vi "TUNA RT main.vi"() -> ()   [LabVIEW 2014]
uses:
  <vilib>/myRIO/Instrument Drivers/Onboard IO/PWM/typedefs/PWM Reference.ctl
  <vilib>/myRIO/Common/Instrument Driver Framework/Utilities/typedefs/myRIO Generic Hardware Reference.ctl
  <vilib>/myRIO/Common/Instrument Driver Framework/Utilities/typedefs/Hardware Version Enum.ctl
  <vilib>/myRIO/Common/Instrument Driver Framework/Utilities/typedefs/myRIO v1.0 Reference.ctl
  <vilib>/myRIO/Common/Instrument Driver Framework/Utilities/typedefs/Generic FPGA Reference.ctl
  <vilib>/myRIO/Common/Instrument Driver Framework/myRIO v1.0/PWM/typedefs/PWM Channels Enum.ctl
  <vilib>/myRIO/Instrument Drivers/Onboard IO/PWM/typedefs/PWM Configuration.ctl
  <vilib>/userdefined/High Color/nirio_resource_hc.ctl
  <vilib>/myRIO/Instrument Drivers/Onboard IO/DIO/typedefs/DIO Reference.ctl
  <vilib>/myRIO/Common/Instrument Driver Framework/myRIO v1.0/DIO/typedefs/DIO Channels List.ctl
  <vilib>/myRIO/Common/Instrument Driver Framework/myRIO v1.0/DIO/typedefs/DIO Channels Enum.ctl
  <vilib>/myRIO/Instrument Drivers/Onboard IO/AI/typedefs/AI Reference.ctl
  <vilib>/myRIO/Common/Instrument Driver Framework/myRIO v1.0/AI/typedefs/AI Channels List.ctl
  <vilib>/myRIO/Common/Instrument Driver Framework/myRIO v1.0/AI/typedefs/AI Channels Enum.ctl
  <vilib>/myRIO/Common/Instrument Driver Framework/Utilities/typedefs/Analog Scaling Constants List.ctl
  <vilib>/myRIO/Common/Instrument Driver Framework/Utilities/typedefs/Analog Scaling Constants.ctl
  <vilib>/Instr/_visa.llb/VISA Flush IO Buffer Mask.ctl
  <vilib>/myRIO/Common/Instrument Driver Framework/myRIO v1.0/PWM/vis/myRIO v1.1 Open PWM.vi
  <vilib>/myRIO/Common/Instrument Driver Framework/myRIO v1.0/DIO/vis/myRIO v1.1 Open DIO.vi
  <vilib>/myRIO/Common/Instrument Driver Framework/myRIO v1.0/AI/vis/myRIO v1.1 Open AI.vi
  <vilib>/myRIO/Common/Instrument Driver Framework/Utilities/vis/Validate Channels.vi
  <vilib>/myRIO/Common/Instrument Driver Framework/myRIO v1.0/PWM/vis/myRIO v1.0 Reserve PWM.vi
  <vilib>/myRIO/Common/Instrument Driver Framework/myRIO v1.0/DIO/vis/myRIO v1.0 Reserve DIO.vi
  <vilib>/myRIO/Common/Instrument Driver Framework/myRIO v1.0/AI/vis/myRIO v1.0 Reserve AI.vi
  <vilib>/myRIO/Common/Instrument Driver Framework/myRIO v1.0/AI/vis/myRIO v1.0 Close AI.vi
  <vilib>/myRIO/Common/Instrument Driver Framework/myRIO v1.0/DIO/vis/myRIO v1.0 Close DIO.vi
  <vilib>/myRIO/Common/Instrument Driver Framework/myRIO v1.0/PWM/vis/myRIO v1.0 Close PWM.vi
  <vilib>/myRIO/Common/Instrument Driver Framework/myRIO v1.0/PWM/vis/myRIO v1.0 Build MUX Configuration PWM.vi
  <vilib>/myRIO/Common/Instrument Driver Framework/myRIO v1.0/Resource Manager/vis/myRIO v1.0 Reserve Channel List.vi
  <vilib>/myRIO/Common/Instrument Driver Framework/myRIO v1.0/DIO/vis/myRIO v1.0 Build MUX Configuration DIO.vi
  <vilib>/myRIO/Common/Instrument Driver Framework/myRIO v1.0/AI/vis/myRIO v1.0 Build MUX Configuration AI.vi
  <vilib>/myRIO/Common/Instrument Driver Framework/myRIO v1.0/AI/vis/myRIO v1.0 Unreserve AI.vi
  <vilib>/myRIO/Common/Instrument Driver Framework/myRIO v1.0/DIO/vis/myRIO v1.0 Unreserve DIO.vi
  <vilib>/myRIO/Common/Instrument Driver Framework/myRIO v1.0/PWM/vis/myRIO v1.0 Unreserve PWM.vi
  <vilib>/myRIO/Common/Instrument Driver Framework/myRIO v1.0/Resource Manager/vis/myRIO v1.0 Create Configuration List.vi
  <vilib>/myRIO/Common/Instrument Driver Framework/myRIO v1.0/Resource Manager/vis/myRIO v1.0 Reserve Channel.vi
  <vilib>/myRIO/Common/Instrument Driver Framework/myRIO v1.0/Resource Manager/vis/myRIO v1.0 Unreserve Channel.vi
  <vilib>/myRIO/Common/Instrument Driver Framework/myRIO v1.0/Resource Manager/vis/myRIO v1.0 Unreserve Channel List.vi
  <vilib>/myRIO/Common/Instrument Driver Framework/myRIO v1.0/Resource Manager/vis/myRIO v1.0 Build Mutex Name.vi
  <vilib>/Utility/VariantDataType/GetNumericInfo.vi
  <vilib>/Utility/error.llb/Error Cluster From Error Code.vi
  <vilib>/myRIO/Common/Instrument Driver Framework/myRIO v1.0/myRIO v1.1 Open.vi
  <vilib>/myRIO/Common/Instrument Driver Framework/myRIO v1.0/AI/vis/myRIO v1.0 Get Scaling Constants AI.vi
  <vilib>/myRIO/Common/Instrument Driver Framework/Utilities/vis/IO Manager.vi
  <vilib>/myRIO/Common/Instrument Driver Framework/Utilities/vis/Configuration Manager.vi
  <vilib>/myRIO/Common/Instrument Driver Framework/myRIO v1.0/myRIO v1.0 Close.vi
  <vilib>/myRIO/Common/Instrument Driver Framework/myRIO v1.0/Resource Manager/vis/myRIO v1.0 Configure IO.vi
  <vilib>/myRIO/Common/Instrument Driver Framework/myRIO v1.0/AI/vis/myRIO v1.0 Read AI.vi
  <vilib>/myRIO/Common/Instrument Driver Framework/myRIO v1.0/DIO/vis/myRIO v1.0 Write DIO.vi
  <vilib>/myRIO/Common/Instrument Driver Framework/myRIO v1.0/PWM/vis/myRIO v1.0 Write PWM.vi
  <vilib>/myRIO/Common/Instrument Driver Framework/myRIO v1.0/DIO/vis/myRIO v1.0 Shutdown DIO.vi
  <vilib>/myRIO/Common/Instrument Driver Framework/myRIO v1.0/PWM/vis/myRIO v1.0 Shutdown PWM.vi
  <vilib>/myRIO/Instrument Drivers/Onboard IO/AI/vis/myRIO AI Open.xnode
  <vilib>/myRIO/Instrument Drivers/Onboard IO/DIO/vis/myRIO DIO Open.xnode
  <vilib>/myRIO/Instrument Drivers/Onboard IO/PWM/vis/myRIO PWM Open.xnode
  <vilib>/myRIO/Instrument Drivers/Onboard IO/AI/AI.lvlib
  <vilib>/myRIO/Instrument Drivers/Onboard IO/DIO/DIO.lvlib
  <vilib>/myRIO/Instrument Drivers/Onboard IO/PWM/PWM.lvlib
panel:
  in  "Tab Control":T1(tab)
  out "GLED":bool
  out "BLED":bool
  out "RLED":bool
  in  "stop":bool
  out "Midbrain?":bool
  out "Rudder":dbl(knob) min=-45.0 max=45.0 step=1.0 scale=-45.0..45.0
  out "Speed":dbl(knob) min=-9.0 max=9.0 step=1.0 scale=-50.0..50.0
  out "Hindbrain?":bool
  out "Forebrain?":bool
  out "Battery Dead?":bool
  out "Complete?":bool=TRUE
  out "Arbiter Graph":cluster{dbl, dbl, dbl[]}(graph)
  out "GPS Time Out?":bool
  in  "Run?":bool
  in  "MSpeed":dbl(slide) scale=-50.0..50.0 scale format="%#.1g"
  in  "MHeading":dbl(slide) scale=-180.0..180.0 scale format="%_1f"
  in  "Manual?":bool
  out "Camera Data":T2(array[cluster])
  out "Boat Status":T3={"GPS"={"X pos"=0, "Y pos"=0, "Heading"=0.0}, "IR Sensors"=[{"Name"="Bow", "Angle"=0.0, "Distance"=0.0}], "MOT BAT"=7.2, "RIO BAT"=7.2}
  out "Act Com":T4
  out "Forebrain ACT":dbl[](array[numeric])
  out "IR Sensors":T5(array[cluster])
  out "GPS":cluster{"X pos":i32, "Y pos":i32, "Heading":dbl}
  out "RED LED":bool
  out "GREEN LED":bool
  out "BLUE LED":bool
  in  "MDF":T6(array[cluster])=[{"Type"=enum."Start", "X"=250, "Y"=250, "Speed"=0, "Behaviors"=enum."Open Water Transit"}, {"Type"=enum."Waypoint", "X"=400, "Y"=100, "Speed"=20, "Behaviors"=enum."P-Wall Follow"}, {"Type"=enum."Waypoint", "X"=250, "Y"=250, "Speed"=20, "Behaviors"=enum."Open Water Transit"}, {"Type"=enum."Waypoint", "X"=250, "Y"=400, "Speed"=20, "Behaviors"=enum."Open Water Transit"}, {"Type"=enum."Waypoint", "X"=100, "Y"=400, "Speed"=20, "Behaviors"=enum."Open Water Transit"}, {"Type"=enum."End", "X"=250, "Y"=250, "Speed"=0, "Behaviors"=enum."Open Water Transit"}]
  in  "TUNA\nTAG":string="C"
  in  "GPS\nerror in":errorcluster
  in  "GPS\nVISA resource name":refnum<visa-resource-name>="ASRL2::INSTR"
  in  "Comms\nVISA resource name":refnum<visa-resource-name>="ASRL1::INSTR"
  in  "Comms\nerror in":errorcluster
  out "Invalid Pos?":bool
  out "error out":errorcluster
  out "Forebrain Comd":T7
  out "Debug IR \nRaw Readings":T5(array[cluster])
  out "Comms\nHandshake?":bool
  out "GPS \nHandshake?":bool
  out "Ready to execute handshake":bool
  out "size(s)":i32
  out "MDF Active":T6(array[cluster])
  # "BEHAVIOR LIGHTS"
  # "To start the Tug, press the \">\" key in the tool bar.\n\nPress the Run? control to start the Mission.\n\nWhen complete the Complete? indicator will light.\n\nIf the Run? is not pressed again, the mission will start again.\n\nAlways press the STOP button to end the operation!!!!!!!!!!!!!"
  # "Press the Manual? button to control\nthe Tug from the sliders"
  # "Stuck indicates that\nthe boat is not moving."
  # "Enter the Letter\nof  your Tug"
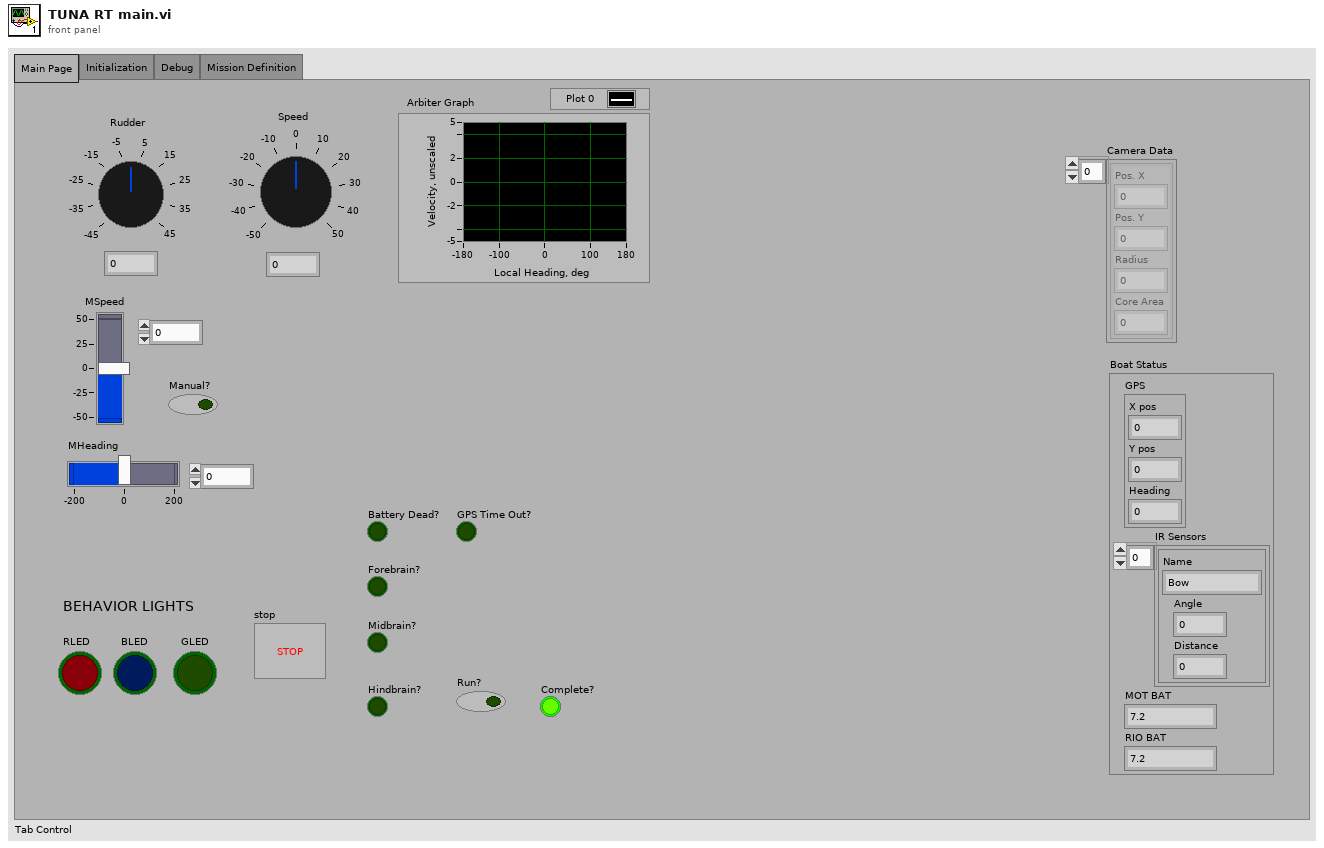
[diagram p1: front panel]
types:
  T1 = enum32{"Main Page", "Initialization", "Debug", "Mission Definition"}
  T2 = cluster{"Pos. X":i32, "Pos. Y":i32, "Radius":i32, "Core Area":i32}[]
  T3 = cluster{"GPS":cluster{"X pos":i32, "Y pos":i32, "Heading":dbl}, "IR Sensors":cluster{"Name":string, "Angle":dbl, "Distance":dbl}[], "MOT BAT":dbl, "RIO BAT":dbl}
  T4 = cluster{"Desired Local\nHeading":dbl, "Desired\nSpeed":dbl}
  T5 = cluster{"Name":string, "Angle":dbl, "Distance":dbl}[]
  T6 = cluster{"Type":enum16{"Start", "Waypoint", "End"}, "X":i32, "Y":i32, "Speed":i32, "Behaviors":enum16{"Open Water Transit", "P-Wall Follow", "S-Wall Follow", "Dock"}}[]
  T7 = cluster{"Behaviors":enum16{"Open Water Transit", "P-Wall Follow", "S-Wall Follow", "Dock"}, "Behavior\nVelocity":dbl}
  T8 = typedef "nirio_resource_hc.ctl" = tag
  T9 = typedef "Hardware Version Enum.ctl" = enum16{"Unknown", "myRIO-1900", "myRIO-1950"}
  T10 = enum16{"Open Water Transit", "P-Wall Follow", "S-Wall Follow", "Dock"}
  T11 = typedef "PWM.lvlib/PWM Reference.ctl" = cluster{"myRIO Reference":T12, "PWM Channels Enum":T15, "PWM Configuration":T16}
  T12 = typedef "myRIO Generic Hardware Reference.ctl" = cluster{"myRIO Model":T9, "myRIO Hardware Reference":T13}
  T13 = typedef "myRIO v1.0 Reference.ctl" = cluster{"Generic FPGA Reference":T14, "Allow multiple opens":bool}
  T14 = typedef "Generic FPGA Reference.ctl" = refnum<k20>
  T15 = typedef "PWM Channels Enum.ctl" = enum16{"Not Connected", "C/PWM0", "C/PWM1", "A/PWM0", "A/PWM1", "A/PWM2", "B/PWM0", "B/PWM1", "B/PWM2"}
  T16 = typedef "PWM.lvlib/PWM Configuration.ctl" = cluster{"Frequency":dbl, "Duty Cycle":dbl}
  T17 = typedef "DIO.lvlib/DIO Reference.ctl" = cluster{"myRIO Reference":T12, "DIO Channels List":T18}
  T18 = typedef "DIO Channels List.ctl" = T19[]
  T19 = typedef "DIO Channels Enum.ctl" = enum16{"Not Connected", "C/DIO0", "C/DIO1", "C/DIO2", "C/DIO3", "C/DIO4", "C/DIO5", "C/DIO6", "C/DIO7", "A/DIO0", "A/DIO1", "A/DIO2", "A/DIO3", "A/DIO4", "A/DIO5", "A/DIO6", "A/DIO7", "A/DIO8", "A/DIO9", "A/DIO10", "A/DIO11", "A/DIO12", "A/DIO13", "A/DIO14", "A/DIO15", "B/DIO0", "B/DIO1", "B/DIO2", "B/DIO3", "B/DIO4", "B/DIO5", "B/DIO6", "B/DIO7", "B/DIO8", "B/DIO9", "B/DIO10", "B/DIO11", "B/DIO12", "B/DIO13", "B/DIO14", "B/DIO15", "LED0", "LED1", "LED2", "LED3", "Button0"}
  T20 = typedef "AI.lvlib/AI Reference.ctl" = cluster{"myRIO Reference":T12, "AI Channels List":T21, "AI Scaling Constants List":T23}
  T21 = typedef "AI Channels List.ctl" = T22[]
  T22 = typedef "AI Channels Enum.ctl" = enum16{"Not Connected", "AudioIn/Left", "AudioIn/Right", "C/AI0", "C/AI1", "A/AI0", "A/AI1", "A/AI2", "A/AI3", "B/AI0", "B/AI1", "B/AI2", "B/AI3"}
  T23 = typedef "Analog Scaling Constants List.ctl" = T24[]
  T24 = typedef "Analog Scaling Constants.ctl" = cluster{"LSB Weight (Volts)":dbl, "Offset (Volts)":dbl, "Signed?":bool}
  T25 = cluster{"Obs Avoid Array":dbl[], "P-Wall Array":dbl[], "S-Wall Array":dbl[], "Unstuck Array":dbl[]}
  T26 = typedef "VISA Flush IO Buffer Mask.ctl" = u16
  T27 = cluster{"Behaviors":enum16{"Open Water Transit", "P-Wall Follow", "S-Wall Follow", "Dock"}, dbl}
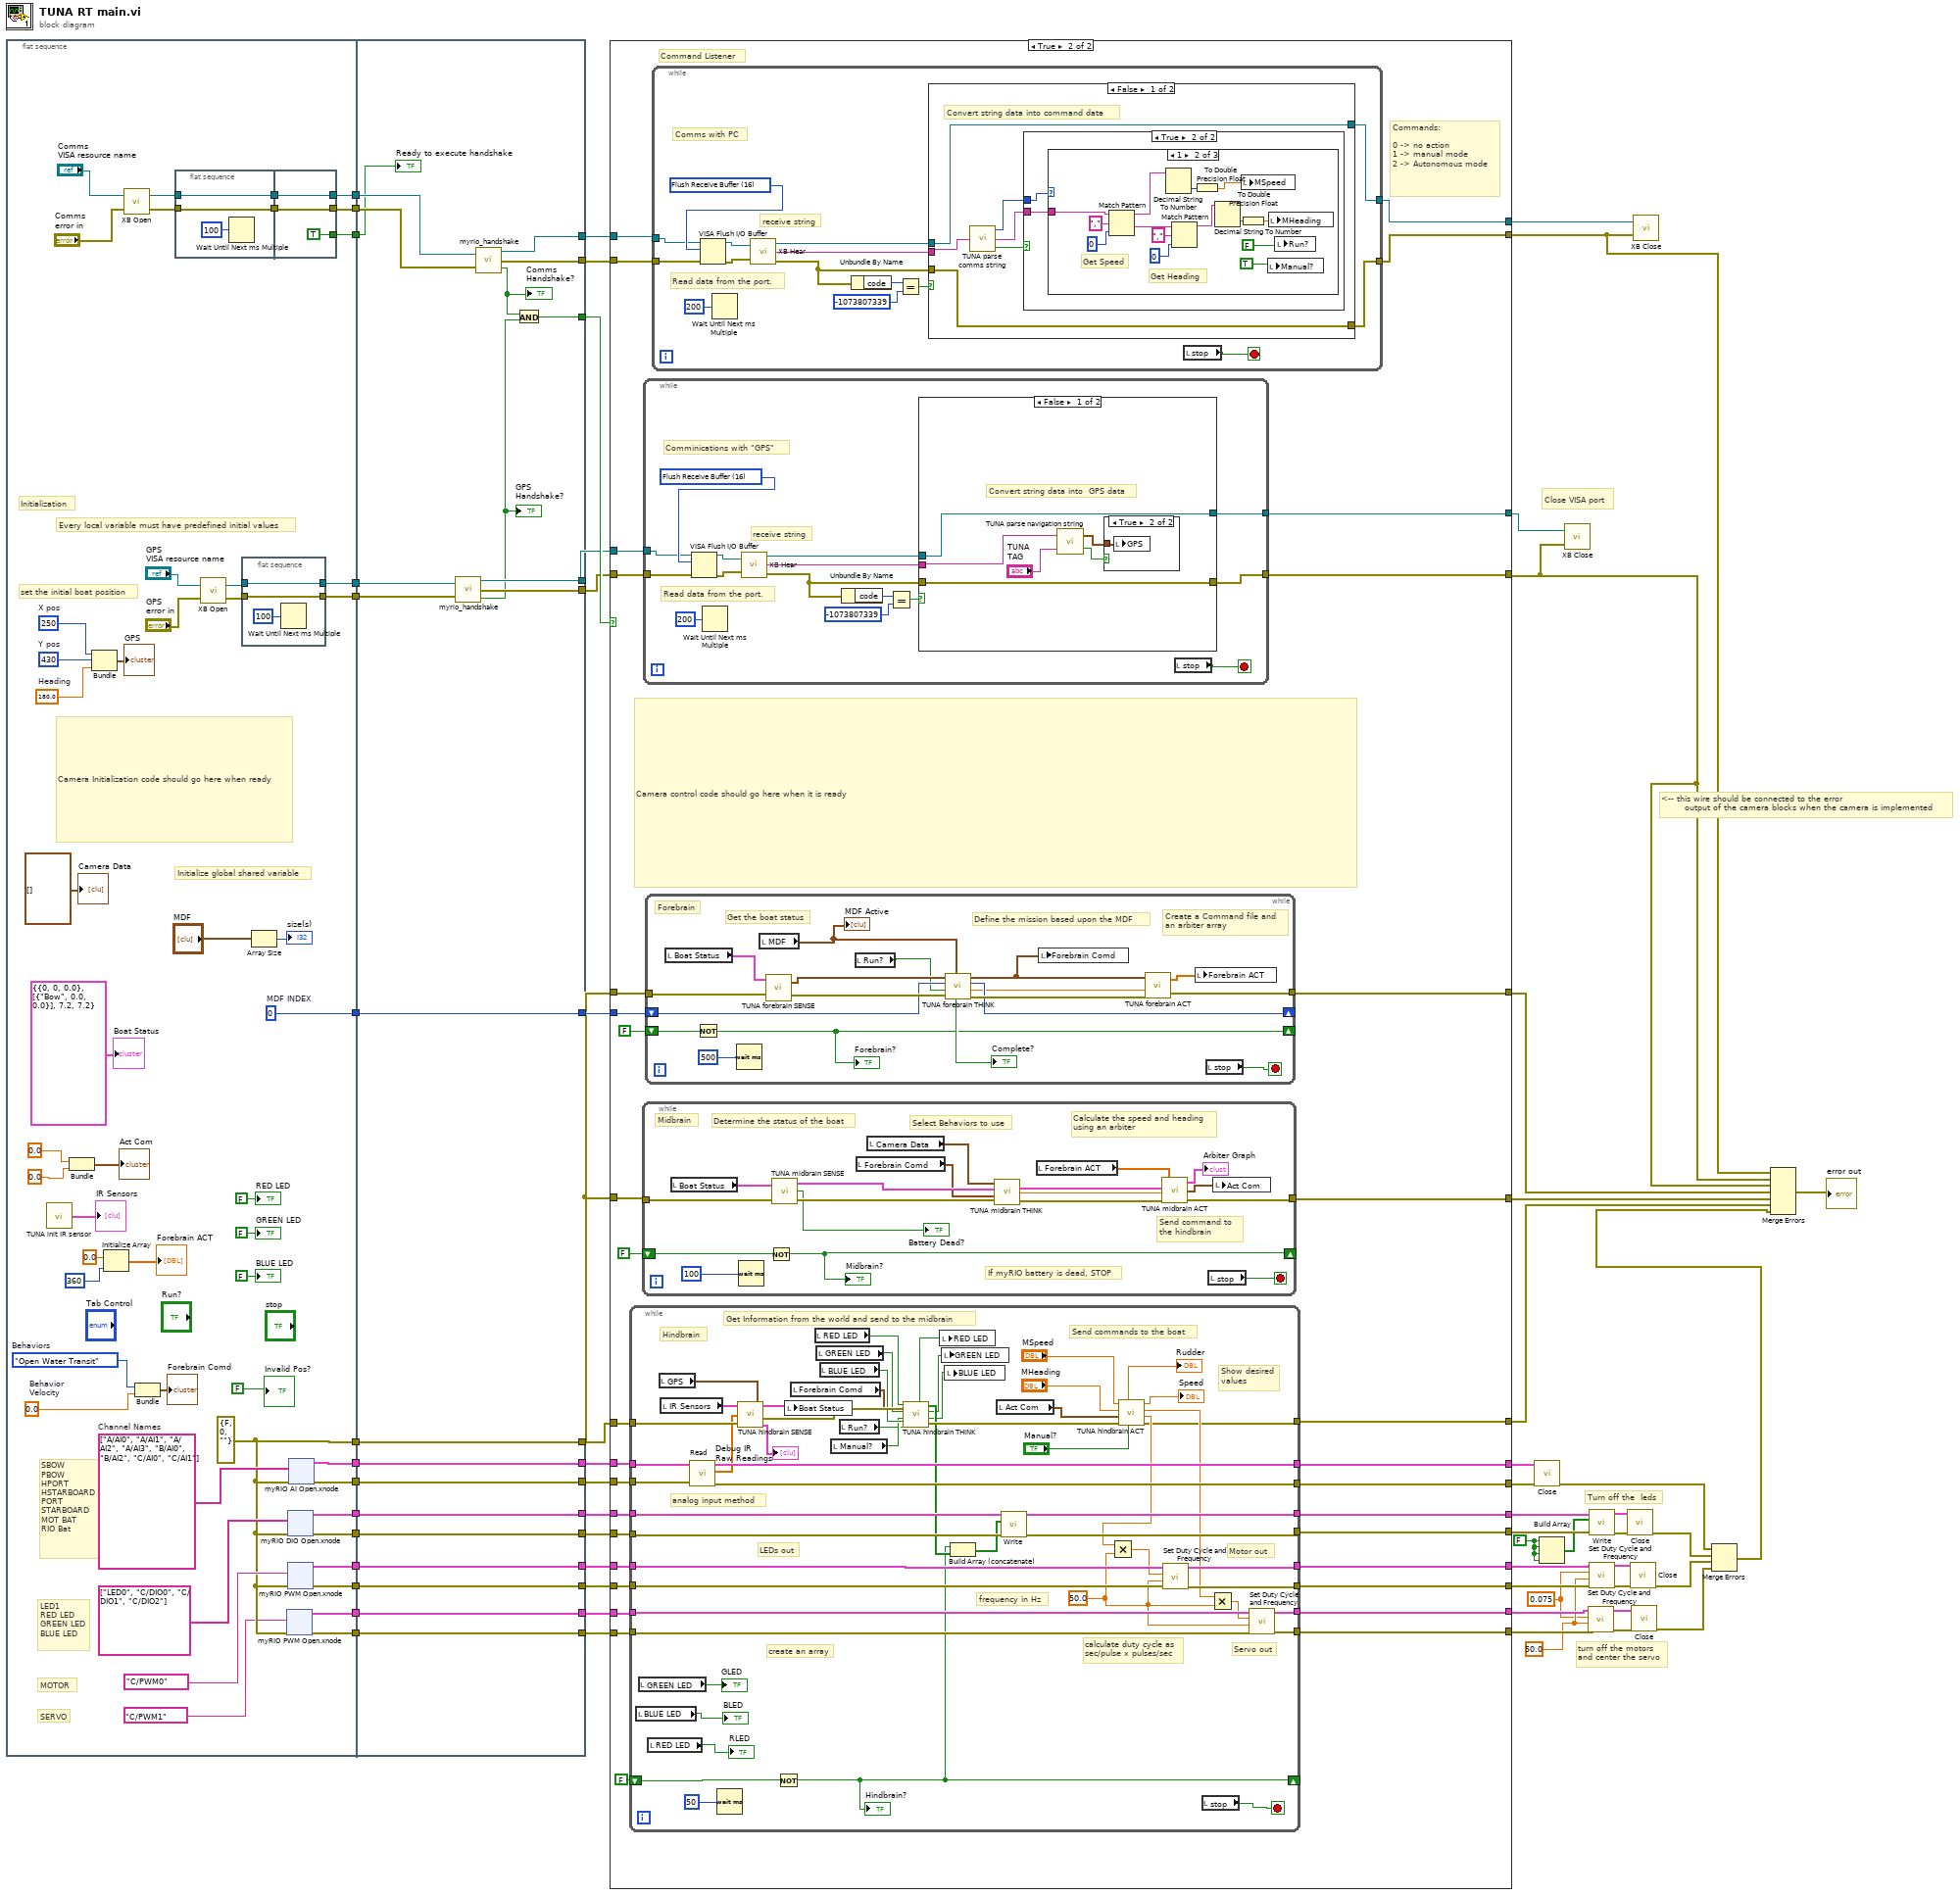
[diagram p0: block diagram]
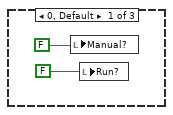
[diagram p4: hidden frame]
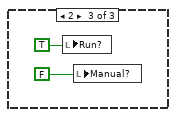
[diagram p5: hidden frame]
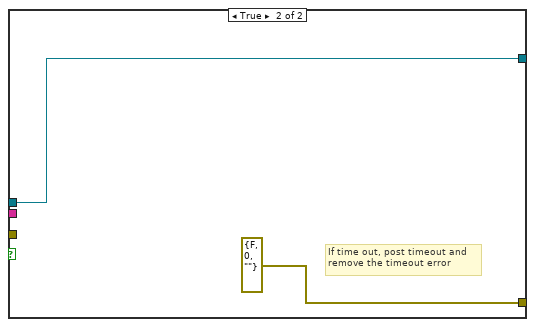
[diagram p6: hidden frame]
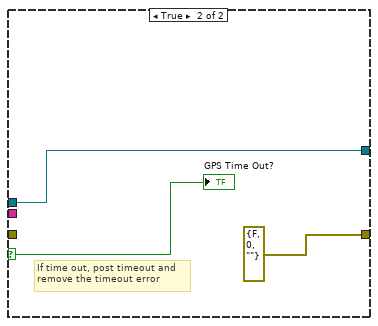
[diagram p8: hidden frame]
diagram:
  w27 = 0.075
  w26 = FALSE
  w28 = 50.0
  # "<-- this wire should be connected to the error\n        output of the camera blocks when the camera is implemented"
  # "Close VISA port"
  # "Turn off the  leds"
  # "turn off the motors\nand center the servo"
  n1 = flat-sequence {
    tunnel: [w88] -> w25
    tunnel: [w104] -> w24
    tunnel: [w96] -> w23
    tunnel: [w95] -> w22
    tunnel: [w93] -> w21
    tunnel: [w92] -> w20
    tunnel: [w90] -> w19
    tunnel: [w89] -> w18
    tunnel: [w86] -> w17
    tunnel: [w85] -> w16
    tunnel: [w69] -> w15
    tunnel: [w70] -> w14
    tunnel: [w72] -> w7
    tunnel: [w71] -> w6
    tunnel: [w62] -> w1
    tunnel: [w200] -> w47
    tunnel: [w201] -> w48
    tunnel: [w202] -> w49
    tunnel: [w203] -> w50
    tunnel: [w204] -> w52
    tunnel: [w205] -> w51
    tunnel: [w206] -> w55
    tunnel: [w207] -> w56
    tunnel: [w208] -> w57
    tunnel: [w209] -> w9
    tunnel: w25 -> [w209]
    tunnel: w24 -> [w208]
    tunnel: w23 -> [w207]
    tunnel: w22 -> [w206]
    tunnel: w21 -> [w205]
    tunnel: w20 -> [w204]
    tunnel: w19 -> [w203]
    tunnel: w18 -> [w202]
    tunnel: w17 -> [w201]
    tunnel: w16 -> [w200]
    tunnel: w15 -> [w199]
    tunnel: w14 -> [w198]
    tunnel: [w197] -> w13
    tunnel: [w196] -> w12
    tunnel: [w195] -> w11
    tunnel: w7 -> [w194]
    tunnel: w6 -> [w193]
    tunnel: [w192] -> w5
    tunnel: [w191] -> w4
    tunnel: w1 -> [w188]
    frame #0 {
      w97 = tag[] ["A/AI0", "A/AI1", "A/AI2", "A/AI3", "B/AI0", "B/AI2", "C/AI0", "C/AI1"]  # Channel Names
      w99 = 430  # Y pos
      w100 = 250  # X pos
      w101 = 180.0  # Heading
      w88 = errorcluster {"status"=FALSE, "code"=0, "source"=""} ("error out")
      w104 = 0  # MDF INDEX
      w108 = 0.0  # Behavior Velocity
      w103 = T10."Open Water Transit"  # Behaviors
      # "Camera Initialization code should go here when ready"
      # "Initialize global shared variable"
      # "LED1\nRED LED\nGREEN LED\nBLUE LED"
      # "SERVO"
      # "MOTOR"
      # "SBOW\nPBOW\nHPORT\nHSTARBOARD\nPORT\nSTARBOARD\nMOT BAT\nRIO Bat"
      # "set the initial boat position"
      # "Every local variable must have predefined initial values"
      # "Initialization"
      n2 = call "TUNA init IR sensor.vi"() -> ("IR Sensors"=→"IR Sensors":T5)  [unwired: 1 in]
      n3 = Bundle(0.0, 0.0) -> (→"Act Com":cluster{dbl, dbl})  [unwired: 1 in]
      n4 = Bundle("X pos"=w100, "Y pos"=w99, "Heading"=w101) -> (→"GPS":cluster{"X pos":i32, "Y pos":i32, "Heading":dbl})  [unwired: 1 in]
      n5 = Initialize Array(0.0 ("element"), 360 ("dimension size")) -> (→"Forebrain ACT":dbl[])
      n6 = call "XB Open.vi"("error in (no error)"="Comms\nerror in", "VISA resource name"="Comms\nVISA resource name") -> ("error out"=w73:errorcluster, "VISA resource name out"=w74:refnum<visa-resource-name>)
      n7 = Bundle("Behaviors"=w103, "Behavior\nVelocity"=w108) -> (→"Forebrain Comd":T7)  [unwired: 1 in]
      n8 = flat-sequence {
        tunnel: w74 -> [w116]
        tunnel: w73 -> [w117]
        tunnel: [w117] -> w64
        tunnel: [w116] -> w63
        tunnel: [w120] -> w72
        tunnel: [w121] -> w71
        tunnel: w64 -> [w121]
        tunnel: w63 -> [w120]
        tunnel: [TRUE] -> w62
        frame #0 {
          n9 = Wait Until Next ms Multiple(millisecond multiple=u32 100) -> ()  [unwired: 1 out]
        }
        frame #1 {
        }
      }
      n10 = call "XB Open.vi"("error in (no error)"="GPS\nerror in", "VISA resource name"="GPS\nVISA resource name") -> ("error out"=w66:errorcluster, "VISA resource name out"=w65:refnum<visa-resource-name>)
      n11 = flat-sequence {
        tunnel: w65 -> [w113]
        tunnel: w66 -> [w114]
        tunnel: [w114] -> w69
        tunnel: [w113] -> w70
        frame #0 {
          n12 = Wait Until Next ms Multiple(millisecond multiple=u32 100) -> ()  [unwired: 1 out]
        }
      }
      n13 = Array Size(array="MDF") -> (size(s)=→"size(s)":i32)
      n14 = xnode "myRIO PWM Open.xnode"("error in (no error)"=w88, "Channel Name"=tag "C/PWM1") -> ("error out"=w86:errorcluster, "PWM Ref Out"=w85:T11)  [unwired: 1 in]
      n15 = xnode "myRIO DIO Open.xnode"("error in (no error)"=w88, "Channel Names"=tag[] ["LED0", "C/DIO0", "C/DIO1", "C/DIO2"]) -> ("error out"=w93:errorcluster, "DIO Ref Out"=w92:T17)  [unwired: 1 in]
      n16 = xnode "myRIO PWM Open.xnode"("error in (no error)"=w88, "Channel Name"=tag "C/PWM0") -> ("error out"=w90:errorcluster, "PWM Ref Out"=w89:T11)  [unwired: 1 in]
      n17 = xnode "myRIO AI Open.xnode"("error in (no error)"=w88, "Channel Names"=w97) -> ("error out"=w96:errorcluster, "AI Ref Out"=w95:T20)  [unwired: 1 in]
      "Invalid Pos?" <- FALSE
      "RED LED" <- FALSE ("RED LED")
      "GREEN LED" <- FALSE ("GREEN LED")
      "BLUE LED" <- FALSE ("WHITE LED")
      "Camera Data" <- T2 [] ("Camera Data")
      "Boat Status" <- T3 {"GPS"={"X pos"=0, "Y pos"=0, "Heading"=0.0}, "IR Sensors"=[{"Name"="Bow", "Angle"=0.0, "Distance"=0.0}], "MOT BAT"=7.2, "RIO BAT"=7.2} ("Boat Status 2")
    }
    frame #1 {
      n18 = call "myrio_handshake.vi"("VISA resource name"=w198, "error in"=w199) -> ("VISA resource name out"=w195:refnum<visa-resource-name>, "error out"=w196:errorcluster, "All Clear \nfrom PC?"=w189:bool)
      "GPS \nHandshake?" <- w189
      n19 = call "myrio_handshake.vi"("VISA resource name"=w194, "error in"=w193) -> ("VISA resource name out"=w191:refnum<visa-resource-name>, "error out"=w192:errorcluster, "All Clear \nfrom PC?"=w190:bool)
      "Comms\nHandshake?" <- w190
      n20 = And(x=w190, y=w189) -> (x .and. y?=w197:bool)
      "Ready to execute handshake" <- w188
    }
  }
  n21 = case shown="True" w13 {
    tunnel: [w213 w255] -> w61
    tunnel: [w213 w254] -> w59
    tunnel: w9 -> [w213 w252]
    tunnel: [w213 w250] -> w58
    tunnel: w57 -> [_ w249]
    tunnel: [w214 w230] -> w8
    tunnel: w56 -> [w216 w248]
    tunnel: w55 -> [w215 w247]
    tunnel: [w216 w246] -> w54
    tunnel: [w215 w245] -> w53
    tunnel: w52 -> [w217 w244]
    tunnel: w51 -> [w218 w243]
    tunnel: w50 -> [w220 w242]
    tunnel: w49 -> [w219 w241]
    tunnel: w48 -> [w222 w240]
    tunnel: w47 -> [w221 w239]
    tunnel: [w222 w238] -> w46
    tunnel: [w221 w237] -> w44
    tunnel: [w220 w236] -> w42
    tunnel: [w219 w235] -> w39
    tunnel: [w218 w234] -> w33
    tunnel: [w217 w233] -> w30
    tunnel: w12 -> [w214 w232]
    tunnel: w11 -> [w212 w231]
    tunnel: [w212 w229] -> w10
    tunnel: w9 -> [_ w227]
    tunnel: w9 -> [_ w228]
    tunnel: w5 -> [w210 w225]
    tunnel: w4 -> [w211 w226]
    tunnel: [w211 w224] -> w3
    tunnel: [w210 w223] -> w2
    frame False {
    }
    frame True {
      # "Commands:\n\n0 -> no action\n1 -> manual mode\n2 -> Autonomous mode"
      # "Command Listener"
      # "Camera control code should go here when it is ready"
      n22 = while {
        tunnel: w252 -> [w393]
        tunnel: [w367] -> w255
        shift-right: [w355] -> _
        shift-left: FALSE -> [w382]
        tunnel: w248 -> [w390]
        tunnel: w247 -> [w389]
        tunnel: [w388] -> w246
        tunnel: [w387] -> w245
        tunnel: w244 -> [w385]
        tunnel: w243 -> [w386]
        tunnel: [w384] -> w234
        tunnel: [w383] -> w233
        tunnel: w242 -> [w380]
        tunnel: w241 -> [w381]
        tunnel: [w379] -> w236
        tunnel: [w378] -> w235
        tunnel: w240 -> [w377]
        tunnel: [w376] -> w238
        tunnel: w239 -> [w375]
        tunnel: [w374] -> w237
        stop <- w395 stop-if-true
        w369 = 50.0
        # "create an array"
        # "frequency in Hz"
        # "calculate duty cycle as\nsec/pulse x pulses/sec"
        # "Show desired\nvalues"
        # "Motor out"
        # "Servo out"
        # "LEDs out"
        # "analog input method"
        # "Send commands to the boat"
        # "Get Information from the world and send to the midbrain"
        # "Hindbrain"
        n23 = local read "BLUE LED"() -> (→"BLED":bool)
        n24 = local read "GREEN LED"() -> (→"GLED":bool)
        n25 = local read "RED LED"() -> (→"RLED":bool)
        n26 = local read "GPS"() -> (w391:cluster{"X pos":i32, "Y pos":i32, "Heading":dbl})
        n27 = local read "IR Sensors"() -> (w353:T5)
        n28 = call <vilib>:"Read.vi"("error in (no error)"=w390, "AI Ref In"=w389) -> ("error out"=w388:errorcluster, "Values"=w373:dbl[], "AI Ref Out"=w387:T20)  [unwired: 7 in]
        n29 = Wait (ms)(milliseconds to wait=u32 50) -> ()  [unwired: 1 out]
        n30 = call "TUNA hindbrain SENSE.vi"("IR Sensors"=w353, "Analog Input Values"=w373, "error in"=w393, "GPS"=w391) -> ("Boat Status"=w354:T3, "error out"=w392:errorcluster, "IR Sensors 2"=→"Debug IR \nRaw Readings":T5)
        n31 = Not(x=w382) -> (.not. x?=w355:bool)
        "Hindbrain?" <- w355
        n32 = local write "Boat Status"(w354) -> ()
        n33 = local read "Forebrain Comd"() -> (w352:T7)
        n34 = local read "RED LED"() -> (w358:bool)
        n35 = local read "GREEN LED"() -> (w357:bool)
        n36 = local read "BLUE LED"() -> (w356:bool)
        n37 = local read "Manual?"() -> (w348:bool)
        n38 = local read "Run?"() -> (w343:bool)
        n39 = call "TUNA hindbrain THINK.vi"("error in"=w392, "BLUE LED"=w356, "Forebrain Comd"=w352, "RUN?"=w343, "MANUAL"=w348, "GREEN LED"=w357, "RED LED"=w358) -> ("error out"=w367:errorcluster, "BLUE LED OUT"=w349:bool, "GREEN LED OUT"=w350:bool, "LED array"=w360:bool[], "RED LED OUT"=w351:bool)
        n40 = local write "RED LED"(w351) -> ()
        n41 = local write "GREEN LED"(w350) -> ()
        n42 = local write "BLUE LED"(w349) -> ()
        n43 = Build Array (concatenate)(w355, w360) -> (w359:bool[])
        n44 = local read "Act Com"() -> (w364:T4)
        n45 = call <vilib>:"Write.vi"("error in (no error)"=w386, "Values"=w359, "DIO Ref In"=w385) -> ("error out"=w384:errorcluster, "DIO Ref Out"=w383:T17)  [unwired: 6 in]
        n46 = call "TUNA hindbrain ACT.vi"("Manual?"="Manual?", "error in"=w367, "Act Com"=w364, "MHeading"="MHeading", "MSpeed"="MSpeed") -> ("Speed"=w372:dbl, "Rudder"=w370:dbl, "Desired\nSpeed"=→"Speed":dbl, "Desired \nRudder"=→"Rudder":dbl)  [unwired: 1 out]
        n47 = Multiply(x=w372, y=w369) -> (x*y=w371:dbl)
        n48 = call <vilib>:"Set Duty Cycle and Frequency.vi"("error in (no error)"=w380, "Frequency [Hz]"=w369, "Duty Cycle"=w371, "PWM Ref In"=w381) -> ("error out"=w379:errorcluster, "PWM Ref Out"=w378:T11)  [unwired: 5 in]
        n49 = local read "stop"() -> (w395:bool)
        n50 = Multiply(x=w370, y=w369) -> (x*y=w368:dbl)
        n51 = call <vilib>:"Set Duty Cycle and Frequency.vi"("error in (no error)"=w377, "Frequency [Hz]"=w369, "Duty Cycle"=w368, "PWM Ref In"=w375) -> ("error out"=w376:errorcluster, "PWM Ref Out"=w374:T11)  [unwired: 5 in]
      }
      n52 = while {
        shift-right: [w401] -> _
        shift-left: FALSE -> [w412]
        tunnel: w227 -> [w411]
        tunnel: [w405] -> w254
        stop <- w413 stop-if-true
        # "If myRIO battery is dead, STOP"
        # "Send command to \nthe hindbrain"
        # "Calculate the speed and heading\nusing an arbiter"
        # "Select Behaviors to use"
        # "Determine the status of the boat"
        # "Midbrain"
        n53 = local read "Boat Status"() -> (w396:T3)
        n54 = Wait (ms)(milliseconds to wait=u32 100) -> ()  [unwired: 1 out]
        n55 = Not(x=w412) -> (.not. x?=w401:bool)
        "Midbrain?" <- w401
        n56 = call "TUNA midbrain SENSE.vi"("Boat Status"=w396, "error in"=w411) -> ("IR Sensors"=w399:T5, "Battery\nDead?"=→"Battery Dead?":bool, "error out"=w409:errorcluster)
        n57 = local read "Forebrain Comd"() -> (w398:T7)
        n58 = local read "Camera Data"() -> (w397:T2)
        n59 = call "TUNA midbrain THINK.vi"("error in"=w409, "Forebrain Comd"=w398, "IR Sensors"=w399, "Camera Data"=w397) -> ("error out"=w408:errorcluster, "Behavior\nVelocity OUT"=w403:dbl, "Behavior arrays"=w406:T25)
        n60 = local read "Forebrain ACT"() -> (w404:dbl[])
        n61 = call "TUNA midbrain ACT.vi"("error in"=w408, "Behavior\nVelocity"=w403, "Behavior arrays"=w406, "Forebrain ACT"=w404) -> ("error out"=w405:errorcluster, "Act Com"=w410:T4, "Waveform Graph"=→"Arbiter Graph":cluster{dbl, dbl, dbl[]})
        n62 = local read "stop"() -> (w413:bool)
        n63 = local write "Act Com"(w410) -> ()
      }
      n64 = while {
        tunnel: w232 -> [w308]
        tunnel: w231 -> [w309]
        tunnel: [w305] -> w230
        tunnel: [w300] -> w229
        stop <- w311 stop-if-true
        w310 = T26 16 items=["Flush Receive Buffer"=16, "Write Transmit Buffer to Device"=32, "Flush Receive Buffer (No I/O)"=64, "Flush Transmit Buffer"=128] ("Mask")
        # "Comminications with \"GPS\""
        # "receive string"
        # "Read data from the port."
        n65 = VISA Flush I/O Buffer(VISA resource name=w309, mask (16)=w310, error in (no error)=w308) -> (VISA resource name out=w307:refnum<visa-resource-name>, error out=w306:errorcluster)
        n66 = Wait Until Next ms Multiple(millisecond multiple=u32 200) -> ()  [unwired: 1 out]
        n67 = call "XB Hear.vi"("VISA resource name"=w307, "error in (no error)"=w306) -> ("VISA resource name out"=w304:refnum<visa-resource-name>, "String Received"=w303:string, "error out"=w301:errorcluster)
        n68 = Unbundle By Name(w301) -> ("code"=w314:i32)
        n69 = Equal?(x=w314, y=-1073807339) -> (x = y?=w302:bool)
        n70 = case shown="False" w302 {
          selector: w302 -> [_ w324]
          tunnel: [w316 errorcluster {"status"=FALSE, "code"=0, "source"=""} ("error out")] -> w305
          tunnel: w304 -> [w318 w323]
          tunnel: w303 -> [w319 _]
          tunnel: [w318 w323] -> w300
          tunnel: w301 -> [w316 _]
          frame False {
            # "Convert string data into  GPS data"
            n71 = call "TUNA parse navigation string.vi"("Header"="TUNA\nTAG", "Nav String"=w319) -> ("Valid?"=w315:bool, "Output GPS"=w317:cluster{"X POS":i32, "Y POS":i32, "HEADING":dbl})
            n72 = case shown="True" w315 {
              tunnel: w317 -> [_ w321]
              frame False {
              }
              frame True {
                n73 = local write "GPS"(w321) -> ()
              }
            }
          }
          frame True {
            # "If time out, post timeout and\nremove the timeout error"
            "GPS Time Out?" <- w324
          }
        }
        n74 = local read "stop"() -> (w311:bool)
      }
      n75 = while {
        tunnel: w228 -> [w340]
        shift-right: [w328] -> _
        shift-left: FALSE -> [w329]
        tunnel: [w337] -> w250
        shift-right: [w333] -> _
        shift-left: w249 -> [w331]
        stop <- w341 stop-if-true
        # "Create a Command file and \nan arbiter array"
        # "Define the mission based upon the MDF"
        # "Get the boat status"
        # "Forebrain"
        n76 = local read "Boat Status"() -> (w335:T3)
        n77 = Not(x=w329) -> (.not. x?=w328:bool)
        "Forebrain?" <- w328
        n78 = Wait (ms)(milliseconds to wait=u32 500) -> ()  [unwired: 1 out]
        n79 = local read "MDF"() -> (w325:T6)
        "MDF Active" <- w325
        n80 = call "TUNA forebrain SENSE.vi"("error in"=w340, "Boat Status"=w335) -> ("error out"=w339:errorcluster, "GPS"=w334:cluster{"X pos":i32, "Y pos":i32, "Heading":dbl})  [unwired: 1 in]
        n81 = local read "Run?"() -> (w327:bool)
        n82 = call "TUNA forebrain THINK.vi"("MDF in"=w325, "error in"=w339, "Run?"=w327, "MDF index"=w331, "GPS"=w334) -> ("error out"=w338:errorcluster, "local Steering\nangle"=w332:dbl, "MDF Index out"=w333:i32, "Behaviors out"=w326:T27, "Complete?"=→"Complete?":bool)
        n83 = local write "Forebrain Comd"(w326) -> ()
        n84 = call "TUNA forebrain ACT.vi"("error in"=w338, "local Steering\nangle"=w332, "Behaviors in"=w326) -> ("error out"=w337:errorcluster, "Forebrain ACT"=w336:dbl[])
        n85 = local write "Forebrain ACT"(w336) -> ()
        n86 = local read "stop"() -> (w341:bool)
      }
      n87 = while {
        tunnel: w225 -> [w265]
        tunnel: w226 -> [w266]
        tunnel: [w262] -> w223
        tunnel: [w257] -> w224
        stop <- w268 stop-if-true
        w267 = T26 16 items=["Flush Receive Buffer"=16, "Write Transmit Buffer to Device"=32, "Flush Receive Buffer (No I/O)"=64, "Flush Transmit Buffer"=128] ("Mask")
        # "Comms with PC"
        # "receive string"
        # "Read data from the port."
        n88 = VISA Flush I/O Buffer(VISA resource name=w266, mask (16)=w267, error in (no error)=w265) -> (VISA resource name out=w264:refnum<visa-resource-name>, error out=w263:errorcluster)
        n89 = Wait Until Next ms Multiple(millisecond multiple=u32 200) -> ()  [unwired: 1 out]
        n90 = call "XB Hear.vi"("VISA resource name"=w264, "error in (no error)"=w263) -> ("VISA resource name out"=w261:refnum<visa-resource-name>, "String Received"=w260:string, "error out"=w258:errorcluster)
        n91 = Unbundle By Name(w258) -> ("code"=w271:i32)
        n92 = Equal?(x=w271, y=-1073807339) -> (x = y?=w259:bool)
        n93 = case shown="False" w259 {
          tunnel: [w276 errorcluster {"status"=FALSE, "code"=0, "source"=""} ("error out")] -> w262
          tunnel: w261 -> [w277 w299]
          tunnel: w260 -> [w275 _]
          tunnel: [w277 w299] -> w257
          tunnel: w258 -> [w276 _]
          frame False {
            # "Convert string data into command data"
            n94 = call "TUNA parse comms string.vi"("Nav String"=w275) -> ("Command Mode"=w272:i32, "command string"=w273:string, "Valid?"=w274:bool)
            n95 = case shown="True" w274 {
              tunnel: w273 -> [_ w278]
              tunnel: w272 -> [_ w279]
              frame False {
              }
              frame True {
                n96 = case shown="1" w279 {
                  tunnel: w278 -> [_ w288 _]
                  frame 0, Default {
                    n97 = local write "Manual?"(FALSE) -> ()
                    n98 = local write "Run?"(FALSE) -> ()
                  }
                  frame 1 {
                    # "Get Heading"
                    # "Get Speed"
                    n99 = Match Pattern(string=w288, regular expression=",", offset (0)=0) -> (before substring=w291:string, after substring=w295:string)  [unwired: 2 out]
                    n100 = Decimal String To Number(string=w291) -> (number=w283:i32)  [unwired: 2 in, 1 out]
                    n101 = Match Pattern(string=w295, regular expression=",", offset (0)=0) -> (before substring=w294:string)  [unwired: 3 out]
                    n102 = To Double Precision Float(number=w283) -> (double precision float=w282:dbl)
                    n103 = Decimal String To Number(string=w294) -> (number=w285:i32)  [unwired: 2 in, 1 out]
                    n104 = local write "MSpeed"(w282) -> ()
                    n105 = To Double Precision Float(number=w285) -> (double precision float=w284:dbl)
                    n106 = local write "Manual?"(TRUE) -> ()
                    n107 = local write "MHeading"(w284) -> ()
                    n108 = local write "Run?"(FALSE) -> ()
                  }
                  frame 2 {
                    n109 = local write "Run?"(TRUE) -> ()
                    n110 = local write "Manual?"(FALSE) -> ()
                  }
                }
              }
            }
          }
          frame True {
            # "If time out, post timeout and\nremove the timeout error"
          }
        }
        n111 = local read "stop"() -> (w268:bool)
      }
    }
  }
  n112 = call <vilib>:"Close.vi"("error in (no error)"=w54, "AI Ref In"=w53) -> ("error out"=w35:errorcluster)  [unwired: 9 in]
  n113 = Build Array(w26, w26, w26, w26) -> (w29:bool[])
  n114 = call "XB Close.vi"("error in (no error)"=w8, "VISA resource name"=w10) -> ()
  n115 = call <vilib>:"Set Duty Cycle and Frequency.vi"("error in (no error)"=w46, "Frequency [Hz]"=w28, "Duty Cycle"=w27, "PWM Ref In"=w44) -> ("error out"=w45:errorcluster, "PWM Ref Out"=w43:T11)  [unwired: 5 in]
  n116 = call <vilib>:"Set Duty Cycle and Frequency.vi"("error in (no error)"=w42, "Frequency [Hz]"=w28, "Duty Cycle"=w27, "PWM Ref In"=w39) -> ("error out"=w41:errorcluster, "PWM Ref Out"=w40:T11)  [unwired: 5 in]
  n117 = call <vilib>:"Write.vi"("error in (no error)"=w33, "Values"=w29, "DIO Ref In"=w30) -> ("error out"=w32:errorcluster, "DIO Ref Out"=w31:T17)  [unwired: 6 in]
  n118 = call <vilib>:"Close.vi"("error in (no error)"=w32, "DIO Ref In"=w31) -> ("error out"=w36:errorcluster)  [unwired: 9 in]
  n119 = call <vilib>:"Close.vi"("error in (no error)"=w41, "PWM Ref In"=w40) -> ("error out"=w37:errorcluster)  [unwired: 9 in]
  n120 = call <vilib>:"Close.vi"("error in (no error)"=w45, "PWM Ref In"=w43) -> ("error out"=w38:errorcluster)  [unwired: 9 in]
  n121 = call "XB Close.vi"("error in (no error)"=w2, "VISA resource name"=w3) -> ()
  n122 = Merge Errors(w35, w36, w37, w38) -> (w34:errorcluster)
  n123 = Merge Errors(w2, w8, w8, w58, w59, w61, w34) -> (→"error out":errorcluster)
